vi "Manage Menu Items.vi"(8 "error in (no error)":errorcluster, 9 "Coords":T1, 10 "CtlRef":refnum<vi>, 11 "Menu in":refnum<k9>) -> (0 "error out":errorcluster)   [LabVIEW 2013, in "Control Addon Shared.lvlib"]
uses:
  <vilib>/Utility/miscctls.llb/LVPoint32TypeDef.ctl
  Control Addon Shared.lvlib
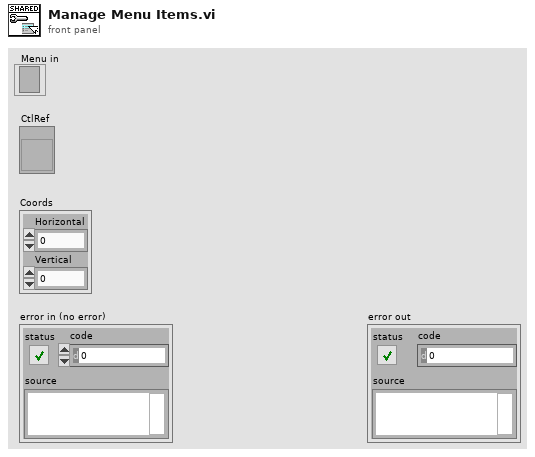
[diagram p1: front panel]
types:
  T1 = typedef "LVPoint32TypeDef.ctl" = cluster{"Horizontal":i32, "Vertical":i32}
  T2 = typedef "LVRowAndColumnTypeDef.ctl" = cluster{"Row":i32, "Column":i32}
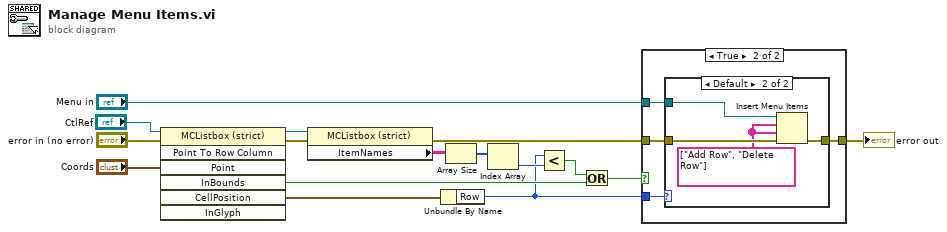
[diagram p0: block diagram]
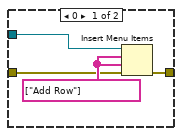
[diagram p3: hidden frame]
diagram:
  n1 = invoke class="MCListbox (strict)" method="Point To Row Column"(reference="CtlRef", error in="error in (no error)", "Point"="Coords") -> (reference out=w9:refnum<vi>, error out=w10:errorcluster, "InBounds"=w14:bool, "CellPosition"=w15:T2)  [unwired: 4 in, 3 out]
  n2 = property class="MCListbox (strict)"(reference=w9, error in=w10) -> (error out=w1:errorcluster, "ItemNames"=w8:string[][])  [unwired: 1 out]
  n3 = Unbundle By Name(w15) -> ("Row"=w5:i32)
  n4 = Array Size(array=w8) -> (size(s)=w7:i32[])
  n5 = Index Array(array=w7) -> (element=w6:i32)  [unwired: 1 in]
  n6 = Less?(x=w5, y=w6) -> (x < y?=w3:bool)
  n7 = Or(x=w3, y=w14) -> (x .or. y?=w4:bool)
  n8 = case shown="True" w4 {
    tunnel: w5 -> [_ w21]
    tunnel: w1 -> [w17 w20]
    tunnel: "Menu in" -> [_ w19]
    tunnel: [w17 w18] -> w16
    frame False {
    }
    frame True {
      n9 = case shown="Default" w21 {
        tunnel: w20 -> [w23 w29]
        tunnel: w19 -> [w22 w28]
        tunnel: [w24 w26] -> w18
        frame 0 {
          w25 = string[] ["Add Row"] ("item names")
          n10 = Insert Menu Items(6:w23, 7:w25, 8:w25, 9:w22) -> (0:w24:errorcluster)  [unwired: 2 in, 2 out]
        }
        frame Default {
          w27 = string[] ["Add Row", "Delete Row"] ("item names")
          n11 = Insert Menu Items(6:w29, 7:w27, 8:w27, 9:w28) -> (0:w26:errorcluster)  [unwired: 2 in, 2 out]
        }
      }
    }
  }
  "error out" <- w16
